vi "Initialize.vi"(7 "Process ID":string, 8 "error in (no error)":errorcluster, 10 "Device Item Ref":T1=18446744073709551615 format="%.0x", 11 "CD_Process in":refnum<class "CD_Process.lvclass">) -> (0 "error out":errorcluster, 3 "CD_Process out":refnum<class "CD_Process.lvclass">)   [LabVIEW 2019, in "TimingDRV Engine.lvlib" / "CD_Process.lvclass"]
uses:
  CD_Process.lvclass
  <vilib>/NI VeriStand/Custom Device API/Custom Device Item Ref.ctl
  TypeDefs/Message.ctl
  TypeDefs/Update.ctl
  CD_Process.lvclass/CD_Process.ctl
  <vilib>/NI VeriStand/Custom Device API/Custom Device API.lvlib
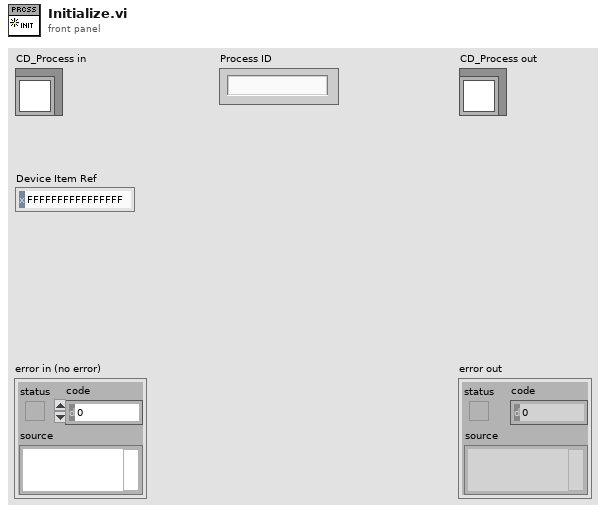
[diagram p1: front panel]
types:
  T1 = typedef "Custom Device API.lvlib/Custom Device Item Ref.ctl" = u64
  T2 = typedef "TimingDRV Engine.lvlib/CD_Process.lvclass/Update.ctl" = cluster{"Update Message":string, "Payload":variant}
  T3 = typedef "TimingDRV Engine.lvlib/CD_Process.lvclass/Message.ctl" = cluster{"Command":string, "Payload":variant}
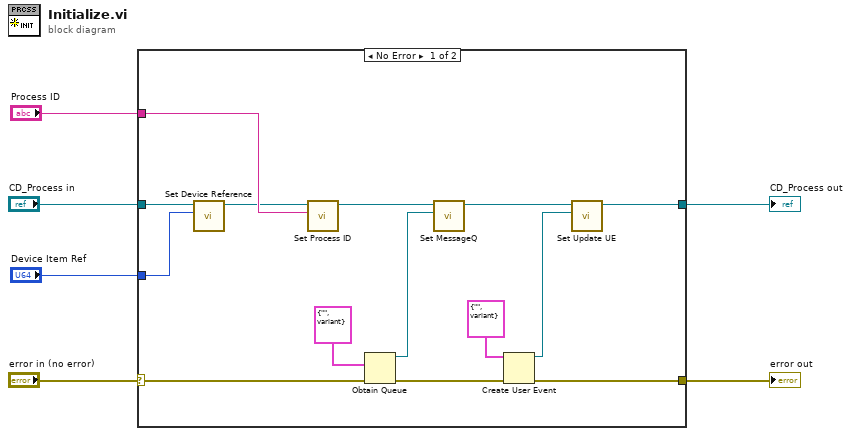
[diagram p0: block diagram]
diagram:
  n1 = case shown="No Error" "error in (no error)" {
    selector: "error in (no error)" -> [w20 w22]
    tunnel: [w11 w22] -> w5
    tunnel: [w10 w21] -> w3
    tunnel: "CD_Process in" -> [w9 w21]
    tunnel: "Process ID" -> [w17 _]
    tunnel: "Device Item Ref" -> [w7 _]
    frame No Error {
      n2 = call "Set Device Reference.vi"("Device Item Ref"=w7, "CD_Process in"=w9) -> ("CD_Process out"=w8:refnum<class "CD_Process.lvclass">)  [unwired: 9 in]
      n3 = call "Set Process ID.vi"("Process ID"=w17, "CD_Process in"=w8) -> ("CD_Process out"=w16:refnum<class "CD_Process.lvclass">)  [unwired: 9 in]
      n4 = Obtain Queue(element data type=T3 {"Command"="", "Payload"=variant}, error in (no error)=w20) -> (queue out=w18:refnum<queue>, error out=w15:errorcluster)  [unwired: 3 in, 1 out]
      n5 = call "Set MessageQ.vi"("MessageQ"=w18, "CD_Process in"=w16) -> ("CD_Process out"=w13:refnum<class "CD_Process.lvclass">)  [unwired: 9 in]
      n6 = Create User Event(user event datatype=T2 {"Update Message"="", "Payload"=variant} ("Update"), error in=w15) -> (user event=w12:refnum<user-event>, error out=w11:errorcluster)
      n7 = call "Set Update UE.vi"("Update UE"=w12, "CD_Process in"=w13) -> ("CD_Process out"=w10:refnum<class "CD_Process.lvclass">)  [unwired: 9 in]
    }
    frame Error {
    }
  }
  "error out" <- w5
  "CD_Process out" <- w3
